vi "LJM_StartInterval.vi"(8 "error in":errorcluster, 10 "Microseconds":i32 format="%.0g", 11 "Interval Handle":i32 format="%.0g") -> (0 "error out":errorcluster)   [LabVIEW 2024]
uses:
  labjackm.dll
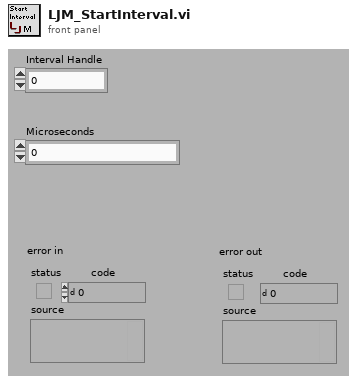
[diagram p1: front panel]
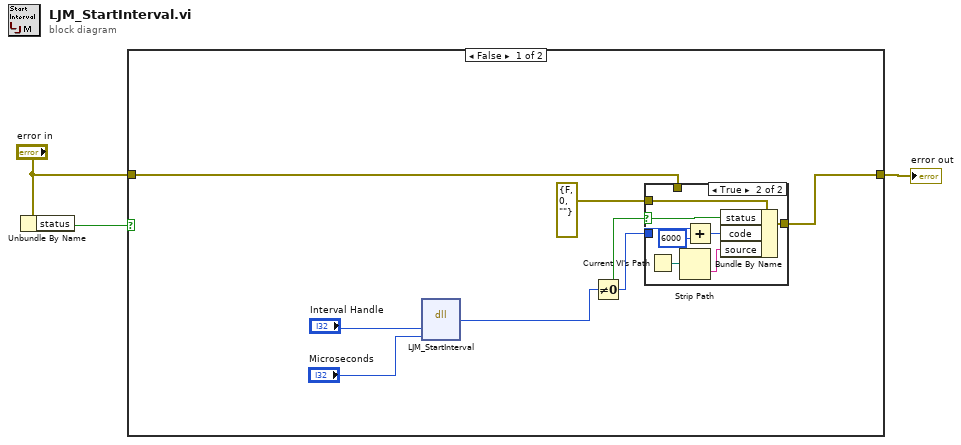
[diagram p0: block diagram]
diagram:
  n1 = Unbundle By Name("error in") -> ("status"=w1:bool)
  n2 = case shown="False" w1 {
    tunnel: "error in" -> [w8 w20]
    tunnel: [w7 w20] -> w3
    frame False {
      n3 = dll-call lib="labjackm.dll" fn="LJM_StartInterval"("IntervalHandle"="Interval Handle", "Microseconds"="Microseconds") -> (w6:i32)  [unwired: 5 in, 2 out]
      n4 = Not Equal To 0?(x=w6) -> (x != 0?=w10:bool)
      n5 = case shown="True" w10 {
        selector: w10 -> [_ w18]
        tunnel: [w11 w19] -> w7
        tunnel: errorcluster {"status"=FALSE, "code"=0, "source"=""} ("error IO") -> [_ w17]
        tunnel: w6 -> [_ w13]
        tunnel: w8 -> [w11 _]
        frame False {
        }
        frame True {
          n6 = Current VI's Path() -> (path=w15:path)
          n7 = Strip Path(path=w15) -> (name=w16:string)  [unwired: 1 out]
          n8 = Add(x=w13, y=6000) -> (x+y=w14:i32)
          n9 = Bundle By Name(cluster=w17, "status"=w18, "code"=w14, "source"=w16) -> (w19:errorcluster)
        }
      }
    }
    frame True {
    }
  }
  "error out" <- w3
